vi "Hide View.vi"(8 "error in (no error)":errorcluster, 11 "ConsoleInterface in":refnum<class "ConsoleSession.lvclass">) -> (0 "error out":errorcluster, 3 "ConsoleInterface out":refnum<class "ConsoleSession.lvclass">)   [LabVIEW 2019, in "ConsoleView.lvlib" / "ConsoleSession.lvclass"]
uses:
  <vilib>/gpm_packages/@cs/event-logger/Source/ConsoleView/ConsoleInterface/ConsoleSession.lvclass
  <vilib>/gpm_packages/@cs/event-logger/Source/Composed Log/Types/MessageCluster.ctl
  <vilib>/gpm_packages/@cs/event-logger/Source/ConsoleView/ConsoleInterface/ConsoleSession.lvclass/ConsoleSession.ctl
  <vilib>/gpm_packages/@cs/event-logger/Source/Composed Log/Composed Log.lvlib
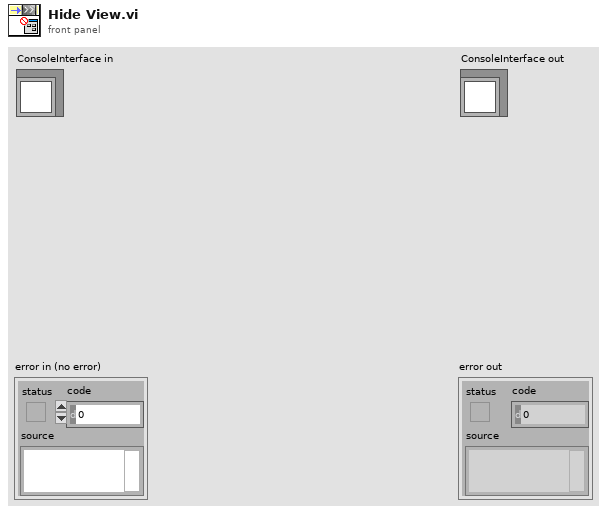
[diagram p1: front panel]
types:
  T1 = typedef "Composed Log.lvlib/MessageCluster.ctl" = cluster{"Message":string, "Data":variant}
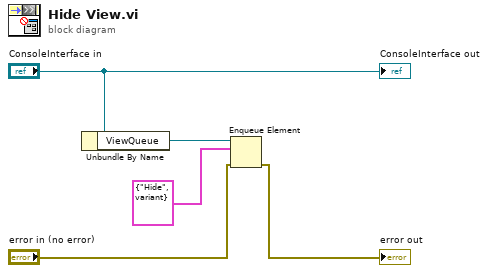
[diagram p0: block diagram]
diagram:
  n1 = Unbundle By Name("ConsoleInterface in") -> ("ViewQueue"=w4:refnum<queue>)
  n2 = Enqueue Element(queue=w4, element=T1 {"Message"="Hide", "Data"=variant}, error in (no error)="error in (no error)") -> (error out=→"error out":errorcluster)  [unwired: 1 in, 2 out]
  "ConsoleInterface out" <- "ConsoleInterface in"
